vi "Disconnect8742.vi"(8 "error in (no error)":errorcluster, 11 "Picomotor8742Comm in":refnum<class "PicoMotor8742Comm.lvclass">) -> (0 "error out":errorcluster, 3 "Picomotor8742Comm out":refnum<class "PicoMotor8742Comm.lvclass">)   [LabVIEW 2020, in "PicoMotor8742Comm.lvclass"]
uses:
  PicoMotor8742Comm.lvclass
  PicoMotor8742Comm.lvclass/PicoMotor8742Comm.ctl
  ASCIICommClass/ASCIICommClass.lvclass
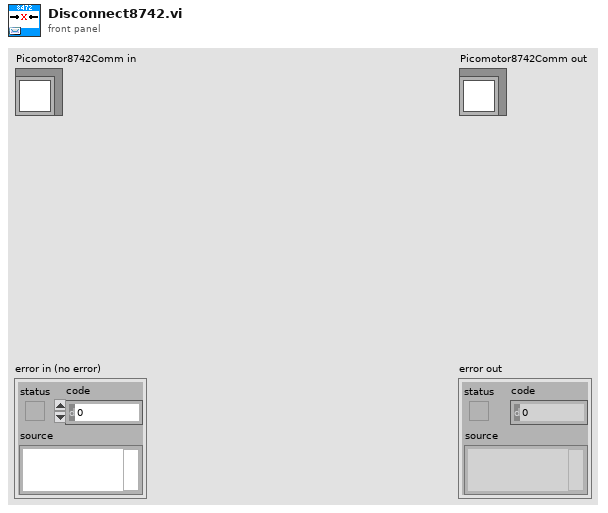
[diagram p1: front panel]
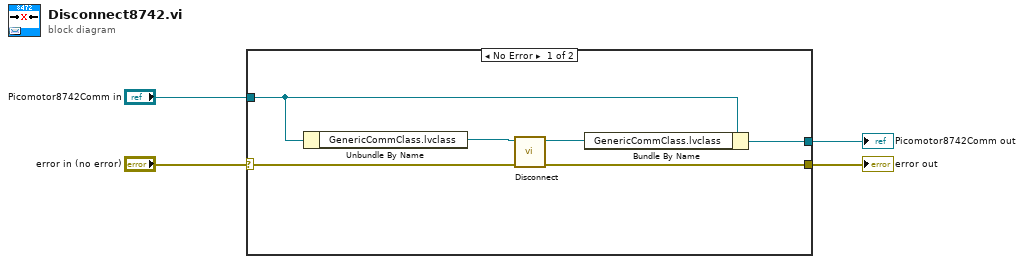
[diagram p0: block diagram]
diagram:
  n1 = case shown="No Error" "error in (no error)" {
    selector: "error in (no error)" -> [w10 w12]
    tunnel: [w9 w12] -> w3
    tunnel: [w5 w11] -> w1
    tunnel: "Picomotor8742Comm in" -> [w6 w11]
    frame No Error {
      n2 = Unbundle By Name(w6) -> ("GenericCommClass.lvclass"=w8:refnum<class "ASCIICommClass.lvclass">)
      n3 = call-dynamic "Disconnect.vi"("error in (no error)"=w10, "StringCommClass in"=w8) -> ("error out"=w9:errorcluster, "StringCommClass out"=w7:refnum<class "ASCIICommClass.lvclass">)  [unwired: 8 in]
      n4 = Bundle By Name(cluster=w6, "GenericCommClass.lvclass"=w7) -> (w5:refnum<class "PicoMotor8742Comm.lvclass">)
    }
    frame Error {
    }
  }
  "error out" <- w3
  "Picomotor8742Comm out" <- w1
